vi "Close MeasurementLink Session.vi"(8 "error in":errorcluster, 9 "initialize and close session behavior":T1, 10 "session in":variant, 11 "session factory in":refnum<class "Session Factory.lvclass">) -> (0 "error out":errorcluster)   [LabVIEW 2021, in "Session Management niSwitch.lvlib" / "Session Factory.lvclass"]
doc: "Closes the local session. If the session represents a remote session, <b>initialize and close session behavior</b> determines whether closing the local session closes the server session or detaches from the server session."
uses:
  Session Factory.lvclass
  Session Factory.lvclass/Session Factory.ctl
  NI Switch_client/NI Switch_client.lvlib
  NI Switch_client/RPC Messages/nidevice_grpc_Session_session/nidevice_grpc_Session_session.lvclass
  NI Switch_client/RPC Messages/nidevice_grpc_Session.ctl
  NI Switch_client/RPC Messages/niswitch_grpc_CloseRequest.ctl
  <vilib>/Plug-In SDKs/Sessions/Instrument/ISession Factory/Initialize and Close Session Behavior.ctl
  <vilib>/Plug-In SDKs/Sessions/Instrument/ISession Factory/ISession Factory.lvclass
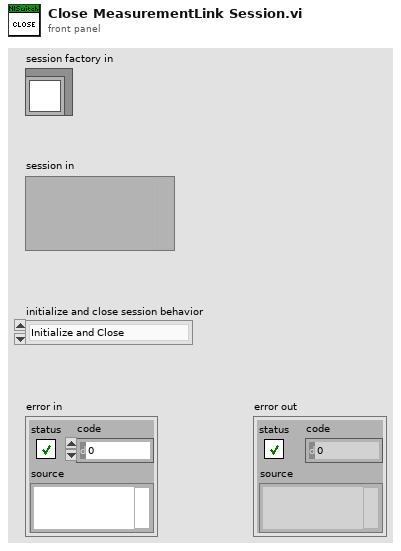
[diagram p1: front panel]
types:
  T1 = typedef "NI Session Management Instrument.lvlib/ISession Factory.lvclass/Initialize and Close Session Behavior.ctl" = enum16{"Initialize and Close", "Attach and Detach", "Initialize and Detach", "Attach and Close"}
  T2 = typedef "NI Switch_client.lvlib/niswitch_grpc_CloseRequest.ctl" = cluster{"vi":T3}
  T3 = typedef "NI Switch_client.lvlib/nidevice_grpc_Session.ctl" = cluster{"nidevice_grpc_Session_session":refnum<class "nidevice_grpc_Session_session.lvclass">}
  T4 = typedef "grpc-lvsupport-release.lvlib/grpcId.ctl" = u64
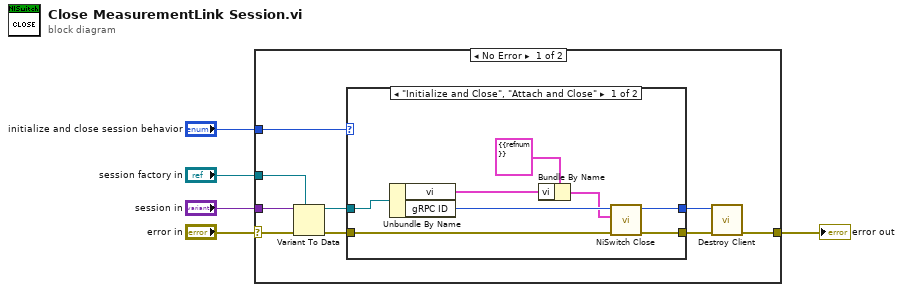
[diagram p0: block diagram]
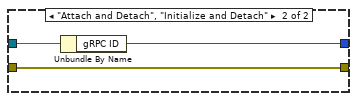
[diagram p2: hidden frame]
diagram:
  n1 = case shown="No Error" "error in" {
    selector: "error in" -> [w12 w26]
    tunnel: [w13 w26] -> w4
    tunnel: "session in" -> [w9 _]
    tunnel: "session factory in" -> [w8 _]
    tunnel: "initialize and close session behavior" -> [w6 _]
    frame No Error {
      n2 = Variant To Data(error in=w12, type=w8, Variant=w9) -> (data=w7:refnum<class "Session Factory.lvclass">, error out=w11:errorcluster)
      n3 = case shown="\"Initialize and Close\", \"Attach and Close\"" w6 {
        tunnel: [w22 w25] -> w14
        tunnel: w11 -> [w21 w25]
        tunnel: [w20 w24] -> w10
        tunnel: w7 -> [w19 w23]
        frame "Initialize and Close", "Attach and Close" {
          n4 = Unbundle By Name(w19) -> ("vi"=w17:T3, "gRPC ID"=w18:T4)
          n5 = Bundle By Name(cluster=T2 {"vi"={"nidevice_grpc_Session_session"=refnum}} ("Request Data"), "vi"=w17) -> (w15:T2)
          n6 = call "NiSwitch Close.vi"("error in"=w21, "Request Data"=w15, "gRPC ID"=w18) -> ("error out"=w22:errorcluster, "gRPC ID out"=w20:T4)  [unwired: 6 in, 1 out]
        }
        frame "Attach and Detach", "Initialize and Detach" {
          n7 = Unbundle By Name(w23) -> ("gRPC ID"=w24:T4)
        }
      }
      n8 = call "Destroy Client.vi"("error in"=w14, "gRPC ID"=w10) -> ("error out"=w13:errorcluster)  [unwired: 9 in]
    }
    frame Error {
    }
  }
  "error out" <- w4
